vi "CumulativeSpectralEnergy.vi"(10 "f.E(f)":dbl[](array[numeric]), 11 "f":dbl[](array[numeric])) -> (2 "plottableBundle":cluster{"X":dbl[], "Array":dbl[]}, 3 "Cumulative Integral":dbl[](array[numeric]))   [LabVIEW 2013]
doc: "Performs a naive rectangular integration- handy for integrating spectra"
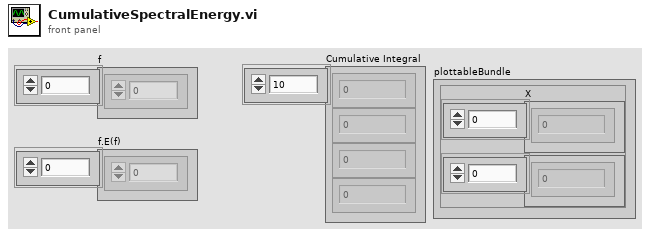
[diagram p1: front panel]
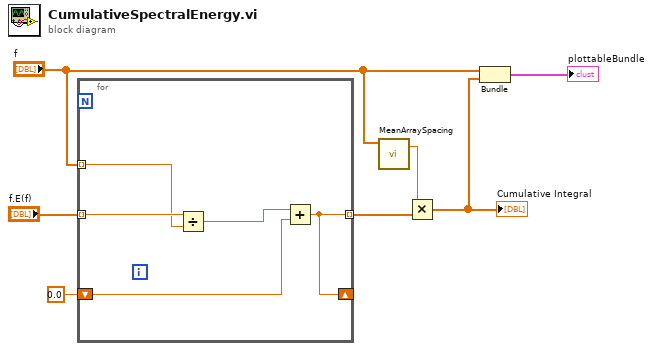
[diagram p0: block diagram]
diagram:
  n1 = for {
    tunnel: "f" -> [w9] mode=indexing
    tunnel: "f.E(f)" -> [w10] mode=indexing
    tunnel: [w11] -> w6 mode=indexing
    shift-right: [w11] -> _
    shift-left: 0.0 -> [w12]
    n2 = Divide(x=w10, y=w9) -> (x/y=w8:dbl)
    n3 = Add(x=w8, y=w12) -> (x+y=w11:dbl)
  }
  n4 = call "MeanArraySpacing.vi"("Array"="f") -> ("Mean Spacing"=w2:dbl)  [unwired: 10 in]
  n5 = Multiply(x=w2, y=w6) -> (x*y=w3:dbl[])
  "Cumulative Integral" <- w3
  n6 = Bundle("f"="f", w3) -> (→"plottableBundle":cluster{"f":dbl[], dbl[]})  [unwired: 1 in]
